vi "PCO_Convert16TOCOL.vi"(0 "ph":u64, 1 "height":i32, 2 "swap_colors":bool=TRUE, 5 "mode":i32, 7 "icolmode":i32, 9 "width":i32, 11 "error in (no error)":errorcluster {"code" format="%x"}, 12 "b16":u16[][](array[numeric])=array1x4097[4097 elements]) -> (4 "ph out":u64, 6 "ErrorMessage":i32 format="%x", 8 "b32":u32[][](array[numeric]), 15 "error out":errorcluster {"code" format="%x"})   [LabVIEW 2020, in "Convert.lvlib"]
doc: "int PCOCONVERT_API PCO_Convert16TOCOL(HANDLE ph, int mode, int icolmode, int width, int height, word *b16, byte *b8);"
uses:
  Convert.lvlib
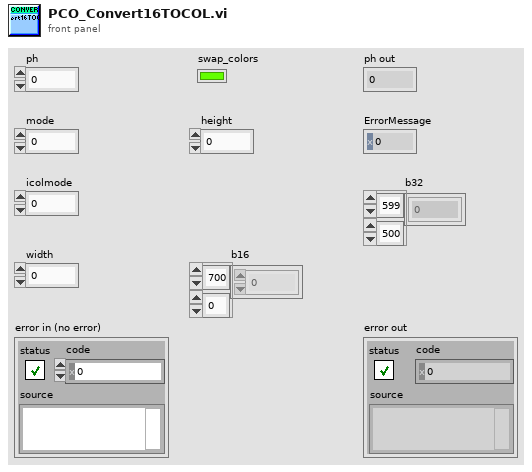
[diagram p1: front panel]
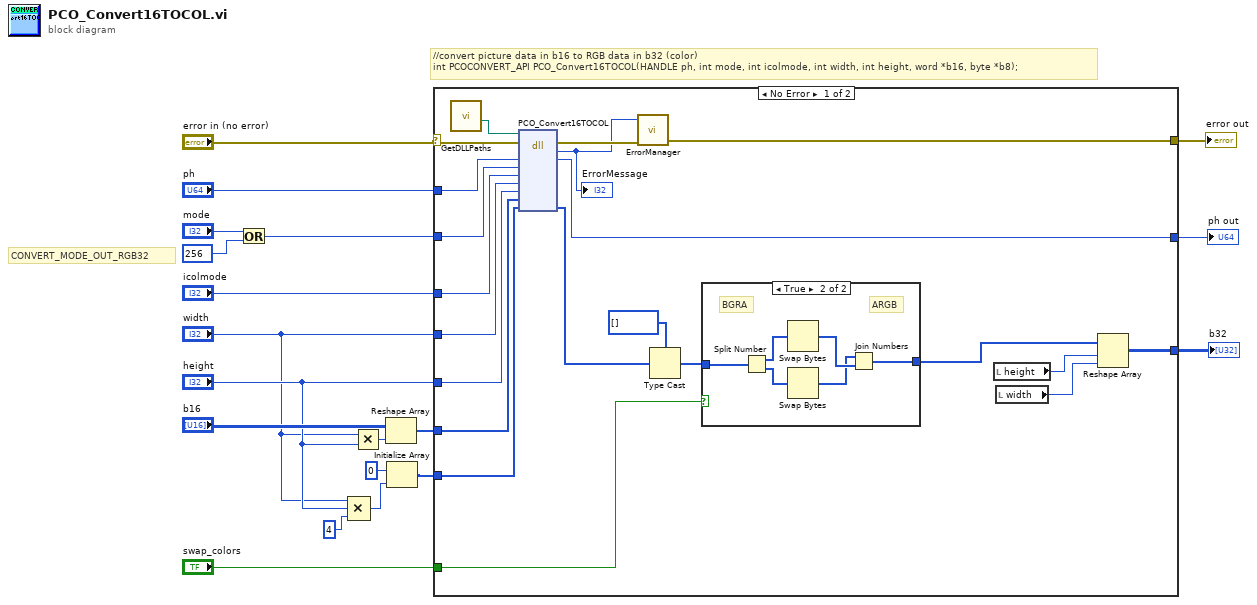
[diagram p0: block diagram]
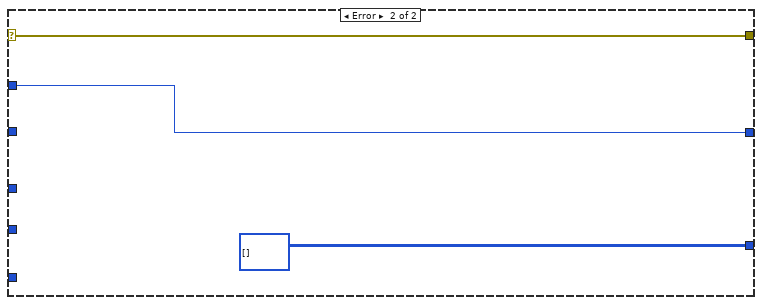
[diagram p3: hidden frame]
diagram:
  # "CONVERT_MODE_OUT_RGB32"
  # "//convert picture data in b16 to RGB data in b32 (color)\nint PCOCONVERT_API PCO_Convert16TOCOL(HANDLE ph, int mode, int icolmode, int width, int height, word *b16, byte *b8);"
  n1 = Or(x="mode", y=256) -> (x .or. y?=w4:i32)
  n2 = Compound Arithmetic op=MULTIPLY("width", "height", 4 ("value")) -> (w13:i32)
  n3 = Multiply(x="width", y="height") -> (x*y=w8:i32)
  n4 = Reshape Array("b16", w8) -> (w11:u16[])
  n5 = Initialize Array(u8 0 ("element"), w13) -> (w15:u8[])
  n6 = case shown="No Error" "error in (no error)" {
    selector: "error in (no error)" -> [w32 w50]
    tunnel: "ph" -> [w40 w49]
    tunnel: [w39 w49] -> w18
    tunnel: w4 -> [w38 _]
    tunnel: "icolmode" -> [w37 _]
    tunnel: "width" -> [w36 _]
    tunnel: "height" -> [w35 _]
    tunnel: w11 -> [w34 _]
    tunnel: [w25 u32[][] [] ("b32")] -> w1
    tunnel: [w30 w50] -> w16
    tunnel: w15 -> [w33 _]
    tunnel: "swap_colors" -> [w20 _]
    frame No Error {
      n7 = call "GetDLLPaths.vi"() -> ("PCO_Conv_Path"=w28:path)  [unwired: 9 in, 2 out]
      n8 = dll-call lib="?" fn="PCO_Convert16TOCOL"(path in=w28, error in=w32, "ph"=w40, "mode"=w38, "icolmode"=w37, "width"=w36, "height"=w35, "b16"=w34, "b8"=w33) -> (error out=w31:errorcluster, "return type"=w29:i32, "ph"=w39:u64, "b8"=w23:u8[])  [unwired: 6 in, 1 out]
      "ErrorMessage" <- w29
      n9 = call "ErrorManager.vi"("error in (no error)"=w31, "error code"=w29) -> ("error out"=w30:errorcluster)  [unwired: 3 in]
      n10 = Type Cast(type=u32[] [] ("b32"), x=w23) -> (*(type *) &x=w22:u32[])
      n11 = case shown="True" w20 {
        tunnel: w22 -> [w41 w47]
        tunnel: [w41 w46] -> w21
        frame False {
        }
        frame True {
          # "ARGB"
          # "BGRA"
          n12 = Split Number(x=w47) -> (hi(x)=w45:u16[], lo(x)=w44:u16[])
          n13 = Swap Bytes(anything=w45) -> (byte swapped=w43:u16[])
          n14 = Swap Bytes(anything=w44) -> (byte swapped=w42:u16[])
          n15 = Join Numbers(hi=w42, lo=w43) -> ((hi.lo)=w46:u32[])
        }
      }
      n16 = local read "height"() -> (w27:i32)
      n17 = local read "width"() -> (w26:i32)
      n18 = Reshape Array(w21, w27, w26) -> (w25:u32[][])
    }
    frame Error {
    }
  }
  "ph out" <- w18
  "b32" <- w1
  "error out" <- w16
